vi "Lin_TransferData.vi"(10 "Seq?":bool, 11 "Data":T1 {"payload" format="%02x"}) -> (3 "Data":T1 {"payload" format="%02x"})   [LabVIEW 2018]
uses:
  Crl/LIN_DataType.ctl
panel:
  # "ms"
  # "ms"
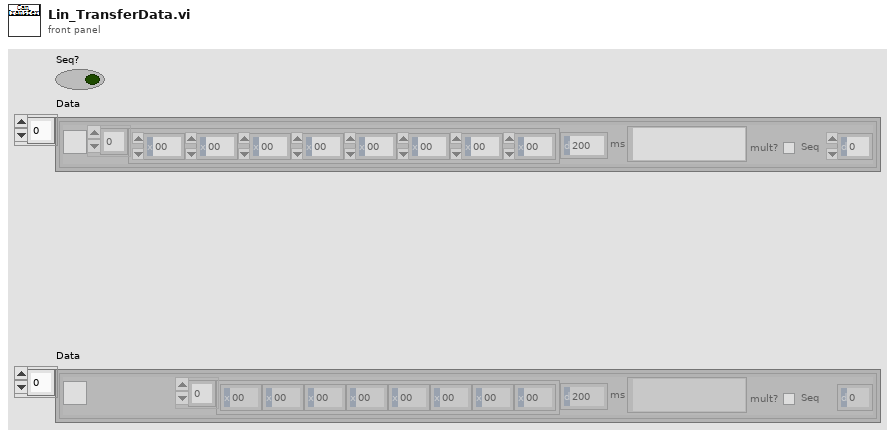
[diagram p1: front panel]
types:
  T1 = typedef "LIN_DataType.ctl" = cluster{"send?":bool, "payload":u8[], "Delays":u32, "Note":string, "mult?":bool, "Seq":i32}[]
  T2 = cluster{"send?":bool, "payload":u8[], "Delays":u32, "Note":string, "mult?":bool, "Seq":i32}[]
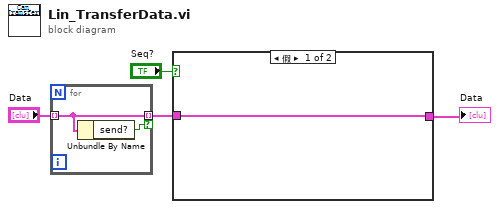
[diagram p0: block diagram]
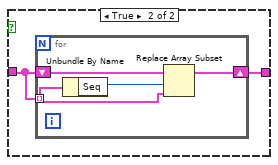
[diagram p2: hidden frame]
diagram:
  n1 = for {
    tunnel: [w5] -> w2 mode=indexing if=w6
    tunnel: "Data" -> [w5] mode=indexing
    n2 = Unbundle By Name(w5) -> ("send?"=w6:bool)
  }
  n3 = case shown="假" "Seq?" {
    tunnel: w2 -> [w7 w9]
    tunnel: [w7 w8] -> w1
    frame False {
    }
    frame True {
      n4 = for {
        tunnel: w9 -> [w11] mode=indexing
        shift-right: [w10] -> w8
        shift-left: w9 -> [w13]
        n5 = Unbundle By Name(w11) -> ("Seq"=w12:i32)
        n6 = Replace Array Subset(array=w13, new element=w11, index=w12) -> (w10:T2)
      }
    }
  }
  "Data" <- w1
